vi "BridgeDirection.vi"(11 "BrickReference in":T1) -> (0 "Direction":bool, 3 "BrickReference out":T1)   [LabVIEW 2012, in "BlockParty4150.lvrbt"]
uses:
  BlockParty4150.lvrbt
  <vilib>/NXT/Subs/LVHSConnector.ctl
  <vilib>/NXT/LegoClasses/BrickReference/BrickReference.lvclass
  <vilib>/NXT/Block Support/NXT_ButtonSelector.ctl
  <vilib>/NXT/Dual Mode Library/Display/drawText.vi
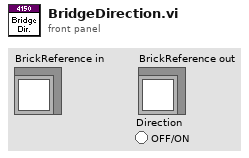
[diagram p1: front panel]
types:
  T1 = typedef "LVHSConnector.ctl" = refnum<class "BrickReference.lvclass">
  T2 = typedef "NXT_ButtonSelector.ctl" = u16
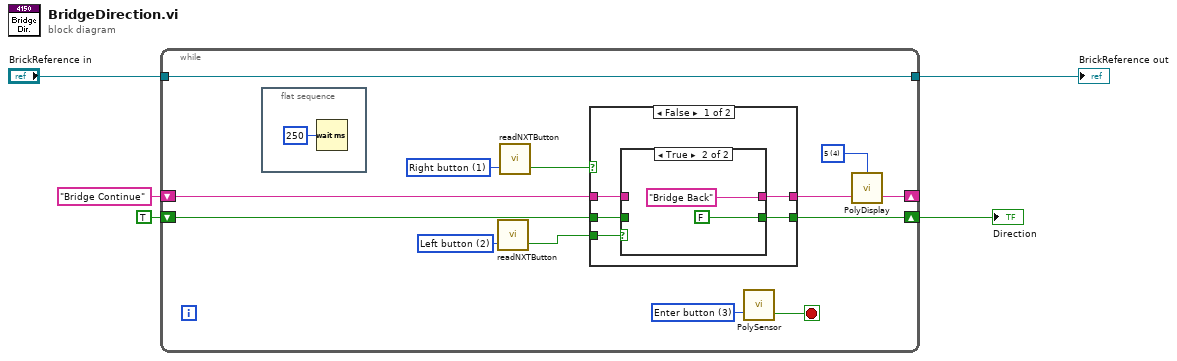
[diagram p0: block diagram]
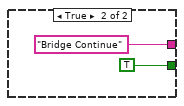
[diagram p3: hidden frame]
diagram:
  n1 = while {
    tunnel: [w17] -> w4
    tunnel: "BrickReference in" -> [w17]
    shift-right: [w8] -> _
    shift-left: "Bridge Continue" -> [w10]
    shift-right: [w6] -> w2
    shift-left: TRUE -> [w9]
    stop <- w15 stop-if-true
    w7 = i16 4 items=["1", "2", "3", "4", "5", "6", "7", "8"] ("Line")
    w11 = T2 1 items=["Enter button"=3, "Left button"=2, "Right button"=1] ("Button (Enter button)")
    w12 = T2 2 items=["Enter button"=3, "Left button"=2, "Right button"=1] ("Button (Enter button)")
    w16 = T2 3 items=["Enter button"=3, "Left button"=2, "Right button"=1] ("Button (Enter button)")
    n2 = flat-sequence {
      frame #0 {
        n3 = Wait (ms)(milliseconds to wait=u32 250) -> ()  [unwired: 1 out]
      }
    }
    n4 = call <vilib>:"readNXTButton.vi"("Button (Enter button)"=w12) -> ("Yes/No"=w14:bool)  [unwired: 2 in, 1 out]
    n5 = call <vilib>:"readNXTButton.vi"("Button (Enter button)"=w11) -> ("Yes/No"=w13:bool)  [unwired: 2 in, 1 out]
    n6 = case shown="False" w13 {
      tunnel: w14 -> [w23 _]
      tunnel: [w22 "Bridge Continue"] -> w8
      tunnel: [w21 TRUE] -> w6
      tunnel: w10 -> [w20 _]
      tunnel: w9 -> [w19 _]
      frame False {
        n7 = case shown="True" w23 {
          tunnel: [w25 "Bridge Back"] -> w22
          tunnel: [w24 FALSE] -> w21
          tunnel: w20 -> [w25 _]
          tunnel: w19 -> [w24 _]
          frame False {
          }
          frame True {
          }
        }
      }
      frame True {
      }
    }
    n8 = call-poly <vilib>:"PolySensor.vi"("Button (Enter button)"=w16) -> ("Yes/No"=w15:bool)  [unwired: 2 in, 1 out]
    n9 = call-poly <vilib>:"PolyDisplay.vi"("Text"=w8, "Line"=w7) -> ()  [unwired: 2 in, 1 out]
  }
  "BrickReference out" <- w4
  "Direction" <- w2
